vi "Test - Draw Teapot.vi"() -> ()   [LabVIEW 2022 SP3, in "Raster.lvlib"] (continued)
"y"=394.73068, "z"=0.98822266}, "UV"={"u"=0.0, "v"=0.0}, "Colour"=12517256}, "Alpha"=0.0, "Alpha Blending Enabled"=FALSE, "Colour"=8630366}, {"Vertex 1"={"Position"={"x"=469.49927, "y"=102.06894, "z"=0.9882263}, "UV"={"u"=0.0, "v"=0.0}, "Colour"=12517256}, "Vertex 2"={"Position"={"x"=448.97742, "y"=109.926476, "z"=0.9887645}, "UV"={"u"=0.0, "v"=0.0}, "Colour"=12517256}, "Vertex 3"={"Position"={"x"=438.67215, "y"=107.464905, "z"=0.9886184}, "UV"={"u"=0.0, "v"=0.0}, "Colour"=12517256}, "Alpha"=0.0, "Alpha Blending Enabled"=FALSE, "Colour"=131841}, {"Vertex 1"={"Position"={"x"=353.4767, "y"=412.15842, "z"=0.988328}, "UV"={"u"=0.0, "v"=0.0}, "Colour"=12517256}, "Vertex 2"={"Position"={"x"=363.17734, "y"=411.41696, "z"=0.9886868}, "UV"={"u"=0.0, "v"=0.0}, "Colour"=12517256}, "Vertex 3"={"Position"={"x"=374.3895, "y"=412.44833, "z"=0.98858166}, "UV"={"u"=0.0, "v"=0.0}, "Colour"=12517256}, "Alpha"=0.0, "Alpha Blending Enabled"=FALSE, "Colour"=9948012}, {"Vertex 1"={"Position"={"x"=272.53372, "y"=105.9543, "z"=0.9882486}, "UV"={"u"=0.0, "v"=0.0}, "Colour"=12517256}, "Vertex 2"={"Position"={"x"=288.70093, "y"=107.824104, "z"=0.9884769}, "UV"={"u"=0.0, "v"=0.0}, "Colour"=12517256}, "Vertex 3"={"Position"={"x"=281.7214, "y"=114.2621, "z"=0.98886466}, "UV"={"u"=0.0, "v"=0.0}, "Colour"=12517256}, "Alpha"=0.0, "Alpha Blending Enabled"=FALSE, "Colour"=131841}, {"Vertex 1"={"Position"={"x"=567.6066, "y"=128.19644, "z"=0.98837066}, "UV"={"u"=0.0, "v"=0.0}, "Colour"=12517256}, "Vertex 2"={"Position"={"x"=574.71216, "y"=132.81842, "z"=0.9882995}, "UV"={"u"=0.0, "v"=0.0}, "Colour"=12517256}, "Vertex 3"={"Position"={"x"=576.8591, "y"=141.4411, "z"=0.98890555}, "UV"={"u"=0.0, "v"=0.0}, "Colour"=12517256}, "Alpha"=0.0, "Alpha Blending Enabled"=FALSE, "Colour"=131841}, {"Vertex 1"={"Position"={"x"=193.75427, "y"=299.13568, "z"=0.9887155}, "UV"={"u"=0.0, "v"=0.0}, "Colour"=12517256}, "Vertex 2"={"Position"={"x"=201.29657, "y"=317.0733, "z"=0.9887643}, "UV"={"u"=0.0, "v"=0.0}, "Colour"=12517256}, "Vertex 3"={"Position"={"x"=202.38127, "y"=318.1235, "z"=0.98807013}, "UV"={"u"=0.0, "v"=0.0}, "Colour"=12517256}, "Alpha"=0.0, "Alpha Blending Enabled"=FALSE, "Colour"=6390341}, {"Vertex 1"={"Position"={"x"=205.55954, "y"=154.37106, "z"=0.98879194}, "UV"={"u"=0.0, "v"=0.0}, "Colour"=12517256}, "Vertex 2"={"Position"={"x"=196.25456, "y"=162.86359, "z"=0.98873174}, "UV"={"u"=0.0, "v"=0.0}, "Colour"=12517256}, "Vertex 3"={"Position"={"x"=197.05006, "y"=154.20059, "z"=0.9880167}, "UV"={"u"=0.0, "v"=0.0}, "Colour"=12517256}, "Alpha"=0.0, "Alpha Blending Enabled"=FALSE, "Colour"=131841}, {"Vertex 1"={"Position"={"x"=546.60223, "y"=113.55681, "z"=0.98858106}, "UV"={"u"=0.0, "v"=0.0}, "Colour"=12517256}, "Vertex 2"={"Position"={"x"=534.80365, "y"=113.363174, "z"=0.98869914}, "UV"={"u"=0.0, "v"=0.0}, "Colour"=12517256}, "Vertex 3"={"Position"={"x"=527.4663, "y"=105.9543, "z"=0.9882486}, "UV"={"u"=0.0, "v"=0.0}, "Colour"=12517256}, "Alpha"=0.0, "Alpha Blending Enabled"=FALSE, "Colour"=131841}, {"Vertex 1"={"Position"={"x"=363.17734, "y"=411.41696, "z"=0.9886868}, "UV"={"u"=0.0, "v"=0.0}, "Colour"=12517256}, "Vertex 2"={"Position"={"x"=353.4767, "y"=412.15842, "z"=0.988328}, "UV"={"u"=0.0, "v"=0.0}, "Colour"=12517256}, "Vertex 3"={"Position"={"x"=341.23203, "y"=410.43784, "z"=0.98850775}, "UV"={"u"=0.0, "v"=0.0}, "Colour"=12517256}, "Alpha"=0.0, "Alpha Blending Enabled"=FALSE, "Colour"=9881963}, {"Vertex 1"={"Position"={"x"=579.84076, "y"=355.96957, "z"=0.98824817}, "UV"={"u"=0.0, "v"=0.0}, "Colour"=12517256}, "Vertex 2"={"Position"={"x"=570.48285, "y"=374.62314, "z"=0.98834187}, "UV"={"u"=0.0, "v"=0.0}, "Colour"=12517256}, "Vertex 3"={"Position"={"x"=572.7935, "y"=370.8628, "z"=0.98893183}, "UV"={"u"=0.0, "v"=0.0}, "Colour"=12517256}, "Alpha"=0.0, "Alpha Blending Enabled"=FALSE, "Colour"=6851402}, {"Vertex 1"={"Position"={"x"=492.24643, "y"=405.47995, "z"=0.98874605}, "UV"={"u"=0.0, "v"=0.0}, "Colour"=12517256}, "Vertex 2"={"Position"={"x"=506.44025, "y"=404.4099, "z"=0.98854554}, "UV"={"u"=0.0, "v"=0.0}, "Colour"=12517256}, "Vertex 3"={"Position"={"x"=496.2093, "y"=407.57056, "z"=0.9881973}, "UV"={"u"=0.0, "v"=0.0}, "Colour"=12517256}, "Alpha"=0.0, "Alpha Blending Enabled"=FALSE, "Colour"=9750378}, {"Vertex 1"={"Position"={"x"=448.97742, "y"=109.926476, "z"=0.9887645}, "UV"={"u"=0.0, "v"=0.0}, "Colour"=12517256}, "Vertex 2"={"Position"={"x"=469.49927, "y"=102.06894, "z"=0.9882263}, "UV"={"u"=0.0, "v"=0.0}, "Colour"=12517256}, "Vertex 3"={"Position"={"x"=481.26578, "y"=106.39749, "z"=0.9884849}, "UV"={"u"=0.0, "v"=0.0}, "Colour"=12517256}, "Alpha"=0.0, "Alpha Blending Enabled"=FALSE, "Colour"=131841}, {"Vertex 1"={"Position"={"x"=598.7034, "y"=317.0733, "z"=0.9887643}, "UV"={"u"=0.0, "v"=0.0}, "Colour"=12517256}, "Vertex 2"={"Position"={"x"=606.2457, "y"=299.13568, "z"=0.9887155}, "UV"={"u"=0.0, "v"=0.0}, "Colour"=12517256}, "Vertex 3"={"Position"={"x"=605.6, "y"=299.08035, "z"=0.98799026}, "UV"={"u"=0.0, "v"=0.0}, "Colour"=12517256}, "Alpha"=0.0, "Alpha Blending Enabled"=FALSE, "Colour"=6390341}, {"Vertex 1"={"Position"={"x"=229.51718, "y"=374.62314, "z"=0.98834187}, "UV"={"u"=0.0, "v"=0.0}, "Colour"=12517256}, "Vertex 2"={"Position"={"x"=220.15924, "y"=355.96957, "z"=0.98824817}, "UV"={"u"=0.0, "v"=0.0}, "Colour"=12517256}, "Vertex 3"={"Position"={"x"=218.2245, "y"=353.0026, "z"=0.9888737}, "UV"={"u"=0.0, "v"=0.0}, "Colour"=12517256}, "Alpha"=0.0, "Alpha Blending Enabled"=FALSE, "Colour"=6851402}, {"Vertex 1"={"Position"={"x"=432.43652, "y"=413.4734, "z"=0.9881905}, "UV"={"u"=0.0, "v"=0.0}, "Colour"=12517256}, "Vertex 2"={"Position"={"x"=425.6105, "y"=412.44833, "z"=0.98858166}, "UV"={"u"=0.0, "v"=0.0}, "Colour"=12517256}, "Vertex 3"={"Position"={"x"=436.8227, "y"=411.41696, "z"=0.9886868}, "UV"={"u"=0.0, "v"=0.0}, "Colour"=12517256}, "Alpha"=0.0, "Alpha Blending Enabled"=FALSE, "Colour"=9948012}, {"Vertex 1"={"Position"={"x"=526.323, "y"=399.39044, "z"=0.9882647}, "UV"={"u"=0.0, "v"=0.0}, "Colour"=12517256}, "Vertex 2"={"Position"={"x"=518.25006, "y"=402.50375, "z"=0.98837876}, "UV"={"u"=0.0, "v"=0.0}, "Colour"=12517256}, "Vertex 3"={"Position"={"x"=525.403, "y"=398.86298, "z"=0.98879325}, "UV"={"u"=0.0, "v"=0.0}, "Colour"=12517256}, "Alpha"=0.0, "Alpha Blending Enabled"=FALSE, "Colour"=10013549}, {"Vertex 1"={"Position"={"x"=511.29907, "y"=107.824104, "z"=0.9884769}, "UV"={"u"=0.0, "v"=0.0}, "Colour"=12517256}, "Vertex 2"={"Position"={"x"=527.4663, "y"=105.9543, "z"=0.9882486}, "UV"={"u"=0.0, "v"=0.0}, "Colour"=12517256}, "Vertex 3"={"Position"={"x"=534.80365, "y"=113.363174, "z"=0.98869914}, "UV"={"u"=0.0, "v"=0.0}, "Colour"=12517256}, "Alpha"=0.0, "Alpha Blending Enabled"=FALSE, "Colour"=131841}, {"Vertex 1"={"Position"={"x"=612.38416, "y"=172.88614, "z"=0.98867583}, "UV"={"u"=0.0, "v"=0.0}, "Colour"=12517256}, "Vertex 2"={"Position"={"x"=603.7455, "y"=162.86359, "z"=0.98873174}, "UV"={"u"=0.0, "v"=0.0}, "Colour"=12517256}, "Vertex 3"={"Position"={"x"=602.9499, "y"=154.20059, "z"=0.9880167}, "UV"={"u"=0.0, "v"=0.0}, "Colour"=12517256}, "Alpha"=0.0, "Alpha Blending Enabled"=FALSE, "Colour"=131841}, {"Vertex 1"={"Position"={"x"=216.54234, "y"=138.55649, "z"=0.9882119}, "UV"={"u"=0.0, "v"=0.0}, "Colour"=12517256}, "Vertex 2"={"Position"={"x"=225.2878, "y"=132.81842, "z"=0.9882995}, "UV"={"u"=0.0, "v"=0.0}, "Colour"=12517256}, "Vertex 3"={"Position"={"x"=223.14096, "y"=141.4411, "z"=0.98890555}, "UV"={"u"=0.0, "v"=0.0}, "Colour"=12517256}, "Alpha"=0.0, "Alpha Blending Enabled"=FALSE, "Colour"=131841}, {"Vertex 1"={"Position"={"x"=471.05533, "y"=410.71017, "z"=0.9881855}, "UV"={"u"=0.0, "v"=0.0}, "Colour"=12517256}, "Vertex 2"={"Position"={"x"=458.76797, "y"=410.43784, "z"=0.98850775}, "UV"={"u"=0.0, "v"=0.0}, "Colour"=12517256}, "Vertex 3"={"Position"={"x"=468.95047, "y"=408.38864, "z"=0.98872197}, "UV"={"u"=0.0, "v"=0.0}, "Colour"=12517256}, "Alpha"=0.0, "Alpha Blending Enabled"=FALSE, "Colour"=9815914}, {"Vertex 1"={"Position"={"x"=496.2093, "y"=407.57056, "z"=0.9881973}, "UV"={"u"=0.0, "v"=0.0}, "Colour"=12517256}, "Vertex 2"={"Position"={"x"=483.04462, "y"=408.23608, "z"=0.98845065}, "UV"={"u"=0.0, "v"=0.0}, "Colour"=12517256}, "Vertex 3"={"Position"={"x"=492.24643, "y"=405.47995, "z"=0.98874605}, "UV"={"u"=0.0, "v"=0.0}, "Colour"=12517256}, "Alpha"=0.0, "Alpha Blending Enabled"=FALSE, "Colour"=9750378}, {"Vertex 1"={"Position"={"x"=344.82437, "y"=98.41171, "z"=0.9880079}, "UV"={"u"=0.0, "v"=0.0}, "Colour"=12517256}, "Vertex 2"={"Position"={"x"=361.32785, "y"=107.464905, "z"=0.9886184}, "UV"={"u"=0.0, "v"=0.0}, "Colour"=12517256}, "Vertex 3"={"Position"={"x"=351.02258, "y"=109.926476, "z"=0.9887645}, "UV"={"u"=0.0, "v"=0.0}, "Colour"=12517256}, "Alpha"=0.0, "Alpha Blending Enabled"=FALSE, "Colour"=131841}, {"Vertex 1"={"Position"={"x"=187.10504, "y"=281.3187, "z"=0.9886726}, "UV"={"u"=0.0, "v"=0.0}, "Colour"=12517256}, "Vertex 2"={"Position"={"x"=193.75427, "y"=299.13568, "z"=0.9887155}, "UV"={"u"=0.0, "v"=0.0}, "Colour"=12517256}, "Vertex 3"={"Position"={"x"=194.40005, "y"=299.08035, "z"=0.98799026}, "UV"={"u"=0.0, "v"=0.0}, "Colour"=12517256}, "Alpha"=0.0, "Alpha Blending Enabled"=FALSE, "Colour"=6126914}, {"Vertex 1"={"Position"={"x"=299.2597, "y"=101.732666, "z"=0.98811007}, "UV"={"u"=0.0, "v"=0.0}, "Colour"=12517256}, "Vertex 2"={"Position"={"x"=318.7342, "y"=106.39749, "z"=0.9884849}, "UV"={"u"=0.0, "v"=0.0}, "Colour"=12517256}, "Vertex 3"={"Position"={"x"=309.68015, "y"=111.224434, "z"=0.9887732}, "UV"={"u"=0.0, "v"=0.0}, "Colour"=12517256}, "Alpha"=0.0, "Alpha Blending Enabled"=FALSE, "Colour"=131841}, {"Vertex 1"={"Position"={"x"=265.19638, "y"=113.363174, "z"=0.98869914}, "UV"={"u"=0.0, "v"=0.0}, "Colour"=12517256}, "Vertex 2"={"Position"={"x"=253.39772, "y"=113.55681, "z"=0.98858106}, "UV"={"u"=0.0, "v"=0.0}, "Colour"=12517256}, "Vertex 3"={"Position"={"x"=260.89398, "y"=105.47977, "z"=0.9880842}, "UV"={"u"=0.0, "v"=0.0}, "Colour"=12517256}, "Alpha"=0.0, "Alpha Blending Enabled"=FALSE, "Colour"=131841}, {"Vertex 1"={"Position"={"x"=574.71216, "y"=132.81842, "z"=0.9882995}, "UV"={"u"=0.0, "v"=0.0}, "Colour"=12517256}, "Vertex 2"={"Position"={"x"=583.45764, "y"=138.55649, "z"=0.9882119}, "UV"={"u"=0.0, "v"=0.0}, "Colour"=12517256}, "Vertex 3"={"Position"={"x"=585.23376, "y"=147.27748, "z"=0.9888514}, "UV"={"u"=0.0, "v"=0.0}, "Colour"=12517256}, "Alpha"=0.0, "Alpha Blending Enabled"=FALSE, "Colour"=131841}, {"Vertex 1"={"Position"={"x"=309.68015, "y"=111.224434, "z"=0.9887732}, "UV"={"u"=0.0, "v"=0.0}, "Colour"=12517256}, "Vertex 2"={"Position"={"x"=288.70093, "y"=107.824104, "z"=0.9884769}, "UV"={"u"=0.0, "v"=0.0}, "Colour"=12517256}, "Vertex 3"={"Position"={"x"=299.2597, "y"=101.732666, "z"=0.98811007}, "UV"={"u"=0.0, "v"=0.0}, "Colour"=12517256}, "Alpha"=0.0, "Alpha Blending Enabled"=FALSE, "Colour"=131841}, {"Vertex 1"={"Position"={"x"=468.95047, "y"=408.38864, "z"=0.98872197}, "UV"={"u"=0.0, "v"=0.0}, "Colour"=12517256}, "Vertex 2"={"Position"={"x"=483.04462, "y"=408.23608, "z"=0.98845065}, "UV"={"u"=0.0, "v"=0.0}, "Colour"=12517256}, "Vertex 3"={"Position"={"x"=471.05533, "y"=410.71017, "z"=0.9881855}, "UV"={"u"=0.0, "v"=0.0}, "Colour"=12517256}, "Alpha"=0.0, "Alpha Blending Enabled"=FALSE, "Colour"=9815914}, {"Vertex 1"={"Position"={"x"=281.74997, "y"=402.50375, "z"=0.98837876}, "UV"={"u"=0.0, "v"=0.0}, "Colour"=12517256}, "Vertex 2"={"Position"={"x"=273.677, "y"=399.39044, "z"=0.9882647}, "UV"={"u"=0.0, "v"=0.0}, "Colour"=12517256}, "Vertex 3"={"Position"={"x"=266.35956, "y"=395.62842, "z"=0.98871076}, "UV"={"u"=0.0, "v"=0.0}, "Colour"=12517256}, "Alpha"=0.0, "Alpha Blending Enabled"=FALSE, "Colour"=10013549}, {"Vertex 1"={"Position"={"x"=196.25456, "y"=162.86359, "z"=0.98873174}, "UV"={"u"=0.0, "v"=0.0}, "Colour"=12517256}, "Vertex 2"={"Position"={"x"=187.61583, "y"=172.88614, "z"=0.98867583}, "UV"={"u"=0.0, "v"=0.0}, "Colour"=12517256}, "Vertex 3"={"Position"={"x"=187.87697, "y"=164.49333, "z"=0.9879249}, "UV"={"u"=0.0, "v"=0.0}, "Colour"=12517256}, "Alpha"=0.0, "Alpha Blending Enabled"=FALSE, "Colour"=131841}, {"Vertex 1"={"Position"={"x"=606.2457, "y"=299.13568, "z"=0.9887155}, "UV"={"u"=0.0, "v"=0.0}, "Colour"=12517256}, "Vertex 2"={"Position"={"x"=612.89496, "y"=281.3187, "z"=0.9886726}, "UV"={"u"=0.0, "v"=0.0}, "Colour"=12517256}, "Vertex 3"={"Position"={"x"=612.6671, "y"=280.0821, "z"=0.98791945}, "UV"={"u"=0.0, "v"=0.0}, "Colour"=12517256}, "Alpha"=0.0, "Alpha Blending Enabled"=FALSE, "Colour"=6126914}, {"Vertex 1"={"Position"={"x"=367.56348, "y"=413.4734, "z"=0.9881905}, "UV"={"u"=0.0, "v"=0.0}, "Colour"=12517256}, "Vertex 2"={"Position"={"x"=374.3895, "y"=412.44833, "z"=0.98858166}, "UV"={"u"=0.0, "v"=0.0}, "Colour"=12517256}, "Vertex 3"={"Position"={"x"=386.75226, "y"=413.1011, "z"=0.988515}, "UV"={"u"=0.0, "v"=0.0}, "Colour"=12517256}, "Alpha"=0.0, "Alpha Blending Enabled"=FALSE, "Colour"=10013805}, {"Vertex 1"={"Position"={"x"=588.9574, "y"=337.11398, "z"=0.98815686}, "UV"={"u"=0.0, "v"=0.0}, "Colour"=12517256}, "Vertex 2"={"Position"={"x"=579.84076, "y"=355.96957, "z"=0.98824817}, "UV"={"u"=0.0, "v"=0.0}, "Colour"=12517256}, "Vertex 3"={"Position"={"x"=581.77545, "y"=353.0026, "z"=0.9888737}, "UV"={"u"=0.0, "v"=0.0}, "Colour"=12517256}, "Alpha"=0.0, "Alpha Blending Enabled"=FALSE, "Colour"=6719817}, {"Vertex 1"={"Position"={"x"=619.56256, "y"=184.55232, "z"=0.98862946}, "UV"={"u"=0.0, "v"=0.0}, "Colour"=12517256}, "Vertex 2"={"Position"={"x"=612.38416, "y"=172.88614, "z"=0.98867583}, "UV"={"u"=0.0, "v"=0.0}, "Colour"=12517256}, "Vertex 3"={"Position"={"x"=612.123, "y"=164.49333, "z"=0.9879249}, "UV"={"u"=0.0, "v"=0.0}, "Colour"=12517256}, "Alpha"=0.0, "Alpha Blending Enabled"=FALSE, "Colour"=131841}, {"Vertex 1"={"Position"={"x"=181.5629, "y"=263.7103, "z"=0.98863673}, "UV"={"u"=0.0, "v"=0.0}, "Colour"=12517256}, "Vertex 2"={"Position"={"x"=187.10504, "y"=281.3187, "z"=0.9886726}, "UV"={"u"=0.0, "v"=0.0}, "Colour"=12517256}, "Vertex 3"={"Position"={"x"=187.33292, "y"=280.0821, "z"=0.98791945}, "UV"={"u"=0.0, "v"=0.0}, "Colour"=12517256}, "Alpha"=0.0, "Alpha Blending Enabled"=FALSE, "Colour"=5731646}, {"Vertex 1"={"Position"={"x"=220.15924, "y"=355.96957, "z"=0.98824817}, "UV"={"u"=0.0, "v"=0.0}, "Colour"=12517256}, "Vertex 2"={"Position"={"x"=211.0426, "y"=337.11398, "z"=0.98815686}, "UV"={"u"=0.0, "v"=0.0}, "Colour"=12517256}, "Vertex 3"={"Position"={"x"=209.52173, "y"=335.05237, "z"=0.9888175}, "UV"={"u"=0.0, "v"=0.0}, "Colour"=12517256}, "Alpha"=0.0, "Alpha Blending Enabled"=FALSE, "Colour"=6719817}, {"Vertex 1"={"Position"={"x"=436.8227, "y"=411.41696, "z"=0.9886868}, "UV"={"u"=0.0, "v"=0.0}, "Colour"=12517256}, "Vertex 2"={"Position"={"x"=446.5233, "y"=412.15842, "z"=0.988328}, "UV"={"u"=0.0, "v"=0.0}, "Colour"=12517256}, "Vertex 3"={"Position"={"x"=432.43652, "y"=413.4734, "z"=0.9881905}, "UV"={"u"=0.0, "v"=0.0}, "Colour"=12517256}, "Alpha"=0.0, "Alpha Blending Enabled"=FALSE, "Colour"=9948012}, {"Vertex 1"={"Position"={"x"=416.8047, "y"=414.309, "z"=0.98810315}, "UV"={"u"=0.0, "v"=0.0}, "Colour"=12517256}, "Vertex 2"={"Position"={"x"=413.24774, "y"=413.1011, "z"=0.988515}, "UV"={"u"=0.0, "v"=0.0}, "Colour"=12517256}, "Vertex 3"={"Position"={"x"=425.6105, "y"=412.44833, "z"=0.98858166}, "UV"={"u"=0.0, "v"=0.0}, "Colour"=12517256}, "Alpha"=0.0, "Alpha Blending Enabled"=FALSE, "Colour"=10013805}, {"Vertex 1"={"Position"={"x"=529.3001, "y"=394.73068, "z"=0.98822266}, "UV"={"u"=0.0, "v"=0.0}, "Colour"=12517256}, "Vertex 2"={"Position"={"x"=526.323, "y"=399.39044, "z"=0.9882647}, "UV"={"u"=0.0, "v"=0.0}, "Colour"=12517256}, "Vertex 3"={"Position"={"x"=533.64044, "y"=395.62842, "z"=0.98871076}, "UV"={"u"=0.0, "v"=0.0}, "Colour"=12517256}, "Alpha"=0.0, "Alpha Blending Enabled"=FALSE, "Colour"=8630366}, {"Vertex 1"={"Position"={"x"=316.9554, "y"=408.23608, "z"=0.98845065}, "UV"={"u"=0.0, "v"=0.0}, "Colour"=12517256}, "Vertex 2"={"Position"={"x"=303.7907, "y"=407.57056, "z"=0.9881973}, "UV"={"u"=0.0, "v"=0.0}, "Colour"=12517256}, "Vertex 3"={"Position"={"x"=293.55975, "y"=404.4099, "z"=0.98854554}, "UV"={"u"=0.0, "v"=0.0}, "Colour"=12517256}, "Alpha"=0.0, "Alpha Blending Enabled"=FALSE, "Colour"=9750378}, {"Vertex 1"={"Position"={"x"=206.8759, "y"=145.61699, "z"=0.9881152}, "UV"={"u"=0.0, "v"=0.0}, "Colour"=12517256}, "Vertex 2"={"Position"={"x"=216.54234, "y"=138.55649, "z"=0.9882119}, "UV"={"u"=0.0, "v"=0.0}, "Colour"=12517256}, "Vertex 3"={"Position"={"x"=214.76619, "y"=147.27748, "z"=0.9888514}, "UV"={"u"=0.0, "v"=0.0}, "Colour"=12517256}, "Alpha"=0.0, "Alpha Blending Enabled"=FALSE, "Colour"=131841}, {"Vertex 1"={"Position"={"x"=612.89496, "y"=281.3187, "z"=0.9886726}, "UV"={"u"=0.0, "v"=0.0}, "Colour"=12517256}, "Vertex 2"={"Position"={"x"=618.4371, "y"=263.7103, "z"=0.98863673}, "UV"={"u"=0.0, "v"=0.0}, "Colour"=12517256}, "Vertex 3"={"Position"={"x"=618.57983, "y"=261.2413, "z"=0.9878602}, "UV"={"u"=0.0, "v"=0.0}, "Colour"=12517256}, "Alpha"=0.0, "Alpha Blending Enabled"=FALSE, "Colour"=5731646}, {"Vertex 1"={"Position"={"x"=554.3064, "y"=114.66924, "z"=0.9885038}, "UV"={"u"=0.0, "v"=0.0}, "Colour"=12517256}, "Vertex 2"={"Position"={"x"=546.60223, "y"=113.55681, "z"=0.98858106}, "UV"={"u"=0.0, "v"=0.0}, "Colour"=12517256}, "Vertex 3"={"Position"={"x"=539.10596, "y"=105.47977, "z"=0.9880842}, "UV"={"u"=0.0, "v"=0.0}, "Colour"=12517256}, "Alpha"=0.0, "Alpha Blending Enabled"=FALSE, "Colour"=131841}, {"Vertex 1"={"Position"={"x"=273.677, "y"=399.39044, "z"=0.9882647}, "UV"={"u"=0.0, "v"=0.0}, "Colour"=12517256}, "Vertex 2"={"Position"={"x"=270.6999, "y"=394.73068, "z"=0.98822266}, "UV"={"u"=0.0, "v"=0.0}, "Colour"=12517256}, "Vertex 3"={"Position"={"x"=263.33197, "y"=391.06378, "z"=0.9886805}, "UV"={"u"=0.0, "v"=0.0}, "Colour"=12517256}, "Alpha"=0.0, "Alpha Blending Enabled"=FALSE, "Colour"=8630366}, {"Vertex 1"={"Position"={"x"=187.61583, "y"=172.88614, "z"=0.98867583}, "UV"={"u"=0.0, "v"=0.0}, "Colour"=12517256}, "Vertex 2"={"Position"={"x"=180.43742, "y"=184.55232, "z"=0.98862946}, "UV"={"u"=0.0, "v"=0.0}, "Colour"=12517256}, "Vertex 3"={"Position"={"x"=180.21684, "y"=176.65451, "z"=0.98784816}, "UV"={"u"=0.0, "v"=0.0}, "Colour"=12517256}, "Alpha"=0.0, "Alpha Blending Enabled"=FALSE, "Colour"=131841}, {"Vertex 1"={"Position"={"x"=341.23203, "y"=410.43784, "z"=0.98850775}, "UV"={"u"=0.0, "v"=0.0}, "Colour"=12517256}, "Vertex 2"={"Position"={"x"=328.94467, "y"=410.71017, "z"=0.9881855}, "UV"={"u"=0.0, "v"=0.0}, "Colour"=12517256}, "Vertex 3"={"Position"={"x"=316.9554, "y"=408.23608, "z"=0.98845065}, "UV"={"u"=0.0, "v"=0.0}, "Colour"=12517256}, "Alpha"=0.0, "Alpha Blending Enabled"=FALSE, "Colour"=9815914}, {"Vertex 1"={"Position"={"x"=248.83113, "y"=403.53403, "z"=0.9885353}, "UV"={"u"=0.0, "v"=0.0}, "Colour"=12517256}, "Vertex 2"={"Position"={"x"=250.87166, "y"=403.82065, "z"=0.98855567}, "UV"={"u"=0.0, "v"=0.0}, "Colour"=12517256}, "Vertex 3"={"Position"={"x"=258.39148, "y"=408.39923, "z"=0.9880488}, "UV"={"u"=0.0, "v"=0.0}, "Colour"=12517256}, "Alpha"=0.0, "Alpha Blending Enabled"=FALSE, "Colour"=9684329}, {"Vertex 1"={"Position"={"x"=455.17563, "y"=98.41171, "z"=0.9880079}, "UV"={"u"=0.0, "v"=0.0}, "Colour"=12517256}, "Vertex 2"={"Position"={"x"=438.67215, "y"=107.464905, "z"=0.9886184}, "UV"={"u"=0.0, "v"=0.0}, "Colour"=12517256}, "Vertex 3"={"Position"={"x"=426.90945, "y"=105.592224, "z"=0.9885072}, "UV"={"u"=0.0, "v"=0.0}, "Colour"=12517256}, "Alpha"=0.0, "Alpha Blending Enabled"=FALSE, "Colour"=131841}, {"Vertex 1"={"Position"={"x"=281.74997, "y"=402.50375, "z"=0.98837876}, "UV"={"u"=0.0, "v"=0.0}, "Colour"=12517256}, "Vertex 2"={"Position"={"x"=293.55975, "y"=404.4099, "z"=0.98854554}, "UV"={"u"=0.0, "v"=0.0}, "Colour"=12517256}, "Vertex 3"={"Position"={"x"=303.7907, "y"=407.57056, "z"=0.9881973}, "UV"={"u"=0.0, "v"=0.0}, "Colour"=12517256}, "Alpha"=0.0, "Alpha Blending Enabled"=FALSE, "Colour"=10014061}, {"Vertex 1"={"Position"={"x"=583.45764, "y"=138.55649, "z"=0.9882119}, "UV"={"u"=0.0, "v"=0.0}, "Colour"=12517256}, "Vertex 2"={"Position"={"x"=593.1241, "y"=145.61699, "z"=0.9881152}, "UV"={"u"=0.0, "v"=0.0}, "Colour"=12517256}, "Vertex 3"={"Position"={"x"=594.4404, "y"=154.37106, "z"=0.98879194}, "UV"={"u"=0.0, "v"=0.0}, "Colour"=12517256}, "Alpha"=0.0, "Alpha Blending Enabled"=FALSE, "Colour"=131841}, {"Vertex 1"={"Position"={"x"=549.12836, "y"=403.82065, "z"=0.98855567}, "UV"={"u"=0.0, "v"=0.0}, "Colour"=12517256}, "Vertex 2"={"Position"={"x"=551.1689, "y"=403.53403, "z"=0.9885353}, "UV"={"u"=0.0, "v"=0.0}, "Colour"=12517256}, "Vertex 3"={"Position"={"x"=543.6329, "y"=408.16522, "z"=0.9880202}, "UV"={"u"=0.0, "v"=0.0}, "Colour"=12517256}, "Alpha"=0.0, "Alpha Blending Enabled"=FALSE, "Colour"=9684329}, {"Vertex 1"={"Position"={"x"=383.19528, "y"=414.309, "z"=0.98810315}, "UV"={"u"=0.0, "v"=0.0}, "Colour"=12517256}, "Vertex 2"={"Position"={"x"=386.75226, "y"=413.1011, "z"=0.988515}, "UV"={"u"=0.0, "v"=0.0}, "Colour"=12517256}, "Vertex 3"={"Position"={"x"=400.0, "y"=413.3279, "z"=0.9884919}, "UV"={"u"=0.0, "v"=0.0}, "Colour"=12517256}, "Alpha"=0.0, "Alpha Blending Enabled"=FALSE, "Colour"=10079597}, {"Vertex 1"={"Position"={"x"=177.34291, "y"=246.40646, "z"=0.98860943}, "UV"={"u"=0.0, "v"=0.0}, "Colour"=12517256}, "Vertex 2"={"Position"={"x"=181.5629, "y"=263.7103, "z"=0.98863673}, "UV"={"u"=0.0, "v"=0.0}, "Colour"=12517256}, "Vertex 3"={"Position"={"x"=181.4201, "y"=261.2413, "z"=0.9878602}, "UV"={"u"=0.0, "v"=0.0}, "Colour"=12517256}, "Alpha"=0.0, "Alpha Blending Enabled"=FALSE, "Colour"=5270329}, {"Vertex 1"={"Position"={"x"=374.3895, "y"=412.44833, "z"=0.98858166}, "UV"={"u"=0.0, "v"=0.0}, "Colour"=12517256}, "Vertex 2"={"Position"={"x"=367.56348, "y"=413.4734, "z"=0.9881905}, "UV"={"u"=0.0, "v"=0.0}, "Colour"=12517256}, "Vertex 3"={"Position"={"x"=353.4767, "y"=412.15842, "z"=0.988328}, "UV"={"u"=0.0, "v"=0.0}, "Colour"=12517256}, "Alpha"=0.0, "Alpha Blending Enabled"=FALSE, "Colour"=9948012}, {"Vertex 1"={"Position"={"x"=400.0, "y"=414.5999, "z"=0.98807275}, "UV"={"u"=0.0, "v"=0.0}, "Colour"=12517256}, "Vertex 2"={"Position"={"x"=400.0, "y"=413.3279, "z"=0.9884919}, "UV"={"u"=0.0, "v"=0.0}, "Colour"=12517256}, "Vertex 3"={"Position"={"x"=413.24774, "y"=413.1011, "z"=0.988515}, "UV"={"u"=0.0, "v"=0.0}, "Colour"=12517256}, "Alpha"=0.0, "Alpha Blending Enabled"=FALSE, "Colour"=10079597}, {"Vertex 1"={"Position"={"x"=624.4671, "y"=197.94992, "z"=0.98859775}, "UV"={"u"=0.0, "v"=0.0}, "Colour"=12517256}, "Vertex 2"={"Position"={"x"=619.56256, "y"=184.55232, "z"=0.98862946}, "UV"={"u"=0.0, "v"=0.0}, "Colour"=12517256}, "Vertex 3"={"Position"={"x"=619.78314, "y"=176.65451, "z"=0.98784816}, "UV"={"u"=0.0, "v"=0.0}, "Colour"=12517256}, "Alpha"=0.0, "Alpha Blending Enabled"=FALSE, "Colour"=461061}, {"Vertex 1"={"Position"={"x"=481.26578, "y"=106.39749, "z"=0.9884849}, "UV"={"u"=0.0, "v"=0.0}, "Colour"=12517256}, "Vertex 2"={"Position"={"x"=500.7403, "y"=101.732666, "z"=0.98811007}, "UV"={"u"=0.0, "v"=0.0}, "Colour"=12517256}, "Vertex 3"={"Position"={"x"=511.29907, "y"=107.824104, "z"=0.9884769}, "UV"={"u"=0.0, "v"=0.0}, "Colour"=12517256}, "Alpha"=0.0, "Alpha Blending Enabled"=FALSE, "Colour"=131841}, {"Vertex 1"={"Position"={"x"=246.46959, "y"=402.33032, "z"=0.9885116}, "UV"={"u"=0.0, "v"=0.0}, "Colour"=12517256}, "Vertex 2"={"Position"={"x"=248.83113, "y"=403.53403, "z"=0.9885353}, "UV"={"u"=0.0, "v"=0.0}, "Colour"=12517256}, "Vertex 3"={"Position"={"x"=256.36713, "y"=408.16522, "z"=0.9880202}, "UV"={"u"=0.0, "v"=0.0}, "Colour"=12517256}, "Alpha"=0.0, "Alpha Blending Enabled"=FALSE, "Colour"=9948012}, {"Vertex 1"={"Position"={"x"=253.39772, "y"=113.55681, "z"=0.98858106}, "UV"={"u"=0.0, "v"=0.0}, "Colour"=12517256}, "Vertex 2"={"Position"={"x"=245.69356, "y"=114.66924, "z"=0.9885038}, "UV"={"u"=0.0, "v"=0.0}, "Colour"=12517256}, "Vertex 3"={"Position"={"x"=253.24971, "y"=106.19928, "z"=0.9879762}, "UV"={"u"=0.0, "v"=0.0}, "Colour"=12517256}, "Alpha"=0.0, "Alpha Blending Enabled"=FALSE, "Colour"=131841}, {"Vertex 1"={"Position"={"x"=618.4371, "y"=263.7103, "z"=0.98863673}, "UV"={"u"=0.0, "v"=0.0}, "Colour"=12517256}, "Vertex 2"={"Position"={"x"=622.6571, "y"=246.40646, "z"=0.98860943}, "UV"={"u"=0.0, "v"=0.0}, "Colour"=12517256}, "Vertex 3"={"Position"={"x"=623.0958, "y"=242.68484, "z"=0.987815}, "UV"={"u"=0.0, "v"=0.0}, "Colour"=12517256}, "Alpha"=0.0, "Alpha Blending Enabled"=FALSE, "Colour"=5270329}, {"Vertex 1"={"Position"={"x"=597.6187, "y"=318.1235, "z"=0.98807013}, "UV"={"u"=0.0, "v"=0.0}, "Colour"=12517256}, "Vertex 2"={"Position"={"x"=588.9574, "y"=337.11398, "z"=0.98815686}, "UV"={"u"=0.0, "v"=0.0}, "Colour"=12517256}, "Vertex 3"={"Position"={"x"=590.4783, "y"=335.05237, "z"=0.9888175}, "UV"={"u"=0.0, "v"=0.0}, "Colour"=12517256}, "Alpha"=0.0, "Alpha Blending Enabled"=FALSE, "Colour"=6587976}, {"Vertex 1"={"Position"={"x"=551.1689, "y"=403.53403, "z"=0.9885353}, "UV"={"u"=0.0, "v"=0.0}, "Colour"=12517256}, "Vertex 2"={"Position"={"x"=553.5304, "y"=402.33032, "z"=0.9885116}, "UV"={"u"=0.0, "v"=0.0}, "Colour"=12517256}, "Vertex 3"={"Position"={"x"=545.9787, "y"=406.98245, "z"=0.98798704}, "UV"={"u"=0.0, "v"=0.0}, "Colour"=12517256}, "Alpha"=0.0, "Alpha Blending Enabled"=FALSE, "Colour"=9948012}, {"Vertex 1"={"Position"={"x"=260.89398, "y"=105.47977, "z"=0.9880842}, "UV"={"u"=0.0, "v"=0.0}, "Colour"=12517256}, "Vertex 2"={"Position"={"x"=272.53372, "y"=105.9543, "z"=0.9882486}, "UV"={"u"=0.0, "v"=0.0}, "Colour"=12517256}, "Vertex 3"={"Position"={"x"=265.19638, "y"=113.363174, "z"=0.98869914}, "UV"={"u"=0.0, "v"=0.0}, "Colour"=12517256}, "Alpha"=0.0, "Alpha Blending Enabled"=FALSE, "Colour"=131841}, {"Vertex 1"={"Position"={"x"=180.43742, "y"=184.55232, "z"=0.98862946}, "UV"={"u"=0.0, "v"=0.0}, "Colour"=12517256}, "Vertex 2"={"Position"={"x"=175.53291, "y"=197.94992, "z"=0.98859775}, "UV"={"u"=0.0, "v"=0.0}, "Colour"=12517256}, "Vertex 3"={"Position"={"x"=174.96338, "y"=190.80173, "z"=0.9877956}, "UV"={"u"=0.0, "v"=0.0}, "Colour"=12517256}, "Alpha"=0.0, "Alpha Blending Enabled"=FALSE, "Colour"=461061}, {"Vertex 1"={"Position"={"x"=328.94467, "y"=410.71017, "z"=0.9881855}, "UV"={"u"=0.0, "v"=0.0}, "Colour"=12517256}, "Vertex 2"={"Position"={"x"=341.23203, "y"=410.43784, "z"=0.98850775}, "UV"={"u"=0.0, "v"=0.0}, "Colour"=12517256}, "Vertex 3"={"Position"={"x"=353.4767, "y"=412.15842, "z"=0.988328}, "UV"={"u"=0.0, "v"=0.0}, "Colour"=12517256}, "Alpha"=0.0, "Alpha Blending Enabled"=FALSE, "Colour"=9882220}, {"Vertex 1"={"Position"={"x"=174.6588, "y"=229.51056, "z"=0.9885921}, "UV"={"u"=0.0, "v"=0.0}, "Colour"=12517256}, "Vertex 2"={"Position"={"x"=177.34291, "y"=246.40646, "z"=0.98860943}, "UV"={"u"=0.0, "v"=0.0}, "Colour"=12517256}, "Vertex 3"={"Position"={"x"=176.9042, "y"=242.68484, "z"=0.987815}, "UV"={"u"=0.0, "v"=0.0}, "Colour"=12517256}, "Alpha"=0.0, "Alpha Blending Enabled"=FALSE, "Colour"=4677427}, {"Vertex 1"={"Position"={"x"=351.02258, "y"=109.926476, "z"=0.9887645}, "UV"={"u"=0.0, "v"=0.0}, "Colour"=12517256}, "Vertex 2"={"Position"={"x"=330.50076, "y"=102.06894, "z"=0.9882263}, "UV"={"u"=0.0, "v"=0.0}, "Colour"=12517256}, "Vertex 3"={"Position"={"x"=344.82437, "y"=98.41171, "z"=0.9880079}, "UV"={"u"=0.0, "v"=0.0}, "Colour"=12517256}, "Alpha"=0.0, "Alpha Blending Enabled"=FALSE, "Colour"=131841}, {"Vertex 1"={"Position"={"x"=211.0426, "y"=337.11398, "z"=0.98815686}, "UV"={"u"=0.0, "v"=0.0}, "Colour"=12517256}, "Vertex 2"={"Position"={"x"=202.38127, "y"=318.1235, "z"=0.98807013}, "UV"={"u"=0.0, "v"=0.0}, "Colour"=12517256}, "Vertex 3"={"Position"={"x"=201.29657, "y"=317.0733, "z"=0.9887643}, "UV"={"u"=0.0, "v"=0.0}, "Colour"=12517256}, "Alpha"=0.0, "Alpha Blending Enabled"=FALSE, "Colour"=6587976}, {"Vertex 1"={"Position"={"x"=622.6571, "y"=246.40646, "z"=0.98860943}, "UV"={"u"=0.0, "v"=0.0}, "Colour"=12517256}, "Vertex 2"={"Position"={"x"=625.34125, "y"=229.51056, "z"=0.9885921}, "UV"={"u"=0.0, "v"=0.0}, "Colour"=12517256}, "Vertex 3"={"Position"={"x"=625.97455, "y"=224.55252, "z"=0.9877862}, "UV"={"u"=0.0, "v"=0.0}, "Colour"=12517256}, "Alpha"=0.0, "Alpha Blending Enabled"=FALSE, "Colour"=4677427}, {"Vertex 1"={"Position"={"x"=243.93146, "y"=400.19006, "z"=0.9884862}, "UV"={"u"=0.0, "v"=0.0}, "Colour"=12517256}, "Vertex 2"={"Position"={"x"=246.46959, "y"=402.33032, "z"=0.9885116}, "UV"={"u"=0.0, "v"=0.0}, "Colour"=12517256}, "Vertex 3"={"Position"={"x"=254.02132, "y"=406.98245, "z"=0.98798704}, "UV"={"u"=0.0, "v"=0.0}, "Colour"=12517256}, "Alpha"=0.0, "Alpha Blending Enabled"=FALSE, "Colour"=9618536}, {"Vertex 1"={"Position"={"x"=626.281, "y"=213.13216, "z"=0.98858607}, "UV"={"u"=0.0, "v"=0.0}, "Colour"=12517256}, "Vertex 2"={"Position"={"x"=624.4671, "y"=197.94992, "z"=0.98859775}, "UV"={"u"=0.0, "v"=0.0}, "Colour"=12517256}, "Vertex 3"={"Position"={"x"=625.0366, "y"=190.80173, "z"=0.9877956}, "UV"={"u"=0.0, "v"=0.0}, "Colour"=12517256}, "Alpha"=0.0, "Alpha Blending Enabled"=FALSE, "Colour"=2437402}, {"Vertex 1"={"Position"={"x"=361.4469, "y"=95.60257, "z"=0.98784006}, "UV"={"u"=0.0, "v"=0.0}, "Colour"=12517256}, "Vertex 2"={"Position"={"x"=373.09055, "y"=105.592224, "z"=0.9885072}, "UV"={"u"=0.0, "v"=0.0}, "Colour"=12517256}, "Vertex 3"={"Position"={"x"=361.32785, "y"=107.464905, "z"=0.9886184}, "UV"={"u"=0.0, "v"=0.0}, "Colour"=12517256}, "Alpha"=0.0, "Alpha Blending Enabled"=FALSE, "Colour"=131841}, {"Vertex 1"={"Position"={"x"=173.71902, "y"=213.13216, "z"=0.98858607}, "UV"={"u"=0.0, "v"=0.0}, "Colour"=12517256}, "Vertex 2"={"Position"={"x"=174.6588, "y"=229.51056, "z"=0.9885921}, "UV"={"u"=0.0, "v"=0.0}, "Colour"=12517256}, "Vertex 3"={"Position"={"x"=174.02547, "y"=224.55252, "z"=0.9877862}, "UV"={"u"=0.0, "v"=0.0}, "Colour"=12517256}, "Alpha"=0.0, "Alpha Blending Enabled"=FALSE, "Colour"=3886890}, {"Vertex 1"={"Position"={"x"=175.53291, "y"=197.94992, "z"=0.98859775}, "UV"={"u"=0.0, "v"=0.0}, "Colour"=12517256}, "Vertex 2"={"Position"={"x"=173.71902, "y"=213.13216, "z"=0.98858607}, "UV"={"u"=0.0, "v"=0.0}, "Colour"=12517256}, "Vertex 3"={"Position"={"x"=173.01648, "y"=206.9948, "z"=0.9877761}, "UV"={"u"=0.0, "v"=0.0}, "Colour"=12517256}, "Alpha"=0.0, "Alpha Blending Enabled"=FALSE, "Colour"=2437402}, {"Vertex 1"={"Position"={"x"=625.34125, "y"=229.51056, "z"=0.9885921}, "UV"={"u"=0.0, "v"=0.0}, "Colour"=12517256}, "Vertex 2"={"Position"={"x"=626.281, "y"=213.13216, "z"=0.98858607}, "UV"={"u"=0.0, "v"=0.0}, "Colour"=12517256}, "Vertex 3"={"Position"={"x"=626.9835, "y"=206.9948, "z"=0.9877761}, "UV"={"u"=0.0, "v"=0.0}, "Colour"=12517256}, "Alpha"=0.0, "Alpha Blending Enabled"=FALSE, "Colour"=3886890}, {"Vertex 1"={"Position"={"x"=553.5304, "y"=402.33032, "z"=0.9885116}, "UV"={"u"=0.0, "v"=0.0}, "Colour"=12517256}, "Vertex 2"={"Position"={"x"=556.06854, "y"=400.19006, "z"=0.9884862}, "UV"={"u"=0.0, "v"=0.0}, "Colour"=12517256}, "Vertex 3"={"Position"={"x"=548.50366, "y"=404.82367, "z"=0.9879514}, "UV"={"u"=0.0, "v"=0.0}, "Colour"=12517256}, "Alpha"=0.0, "Alpha Blending Enabled"=FALSE, "Colour"=9618536}, {"Vertex 1"={"Position"={"x"=558.6956, "y"=116.502, "z"=0.9884599}, "UV"={"u"=0.0, "v"=0.0}, "Colour"=12517256}, "Vertex 2"={"Position"={"x"=554.3064, "y"=114.66924, "z"=0.9885038}, "UV"={"u"=0.0, "v"=0.0}, "Colour"=12517256}, "Vertex 3"={"Position"={"x"=546.75024, "y"=106.19928, "z"=0.9879762}, "UV"={"u"=0.0, "v"=0.0}, "Colour"=12517256}, "Alpha"=0.0, "Alpha Blending Enabled"=FALSE, "Colour"=131841}, {"Vertex 1"={"Position"={"x"=197.05006, "y"=154.20059, "z"=0.9880167}, "UV"={"u"=0.0, "v"=0.0}, "Colour"=12517256}, "Vertex 2"={"Position"={"x"=206.8759, "y"=145.61699, "z"=0.9881152}, "UV"={"u"=0.0, "v"=0.0}, "Colour"=12517256}, "Vertex 3"={"Position"={"x"=205.55954, "y"=154.37106, "z"=0.98879194}, "UV"={"u"=0.0, "v"=0.0}, "Colour"=12517256}, "Alpha"=0.0, "Alpha Blending Enabled"=FALSE, "Colour"=131841}, {"Vertex 1"={"Position"={"x"=527.4663, "y"=105.9543, "z"=0.9882486}, "UV"={"u"=0.0, "v"=0.0}, "Colour"=12517256}, "Vertex 2"={"Position"={"x"=539.10596, "y"=105.47977, "z"=0.9880842}, "UV"={"u"=0.0, "v"=0.0}, "Colour"=12517256}, "Vertex 3"={"Position"={"x"=546.60223, "y"=113.55681, "z"=0.98858106}, "UV"={"u"=0.0, "v"=0.0}, "Colour"=12517256}, "Alpha"=0.0, "Alpha Blending Enabled"=FALSE, "Colour"=131841}, {"Vertex 1"={"Position"={"x"=506.44025, "y"=404.4099, "z"=0.98854554}, "UV"={"u"=0.0, "v"=0.0}, "Colour"=12517256}, "Vertex 2"={"Position"={"x"=518.25006, "y"=402.50375, "z"=0.98837876}, "UV"={"u"=0.0, "v"=0.0}, "Colour"=12517256}, "Vertex 3"={"Position"={"x"=507.2441, "y"=405.96255, "z"=0.9879849}, "UV"={"u"=0.0, "v"=0.0}, "Colour"=12517256}, "Alpha"=0.0, "Alpha Blending Enabled"=FALSE, "Colour"=10014061}, {"Vertex 1"={"Position"={"x"=241.36343, "y"=397.0934, "z"=0.9884605}, "UV"={"u"=0.0, "v"=0.0}, "Colour"=12517256}, "Vertex 2"={"Position"={"x"=243.93146, "y"=400.19006, "z"=0.9884862}, "UV"={"u"=0.0, "v"=0.0}, "Colour"=12517256}, "Vertex 3"={"Position"={"x"=251.49637, "y"=404.82367, "z"=0.9879514}, "UV"={"u"=0.0, "v"=0.0}, "Colour"=12517256}, "Alpha"=0.0, "Alpha Blending Enabled"=FALSE, "Colour"=9025634}, {"Vertex 1"={"Position"={"x"=245.69356, "y"=114.66924, "z"=0.9885038}, "UV"={"u"=0.0, "v"=0.0}, "Colour"=12517256}, "Vertex 2"={"Position"={"x"=241.30443, "y"=116.502, "z"=0.9884599}, "UV"={"u"=0.0, "v"=0.0}, "Colour"=12517256}, "Vertex 3"={"Position"={"x"=248.879, "y"=107.86597, "z"=0.98791444}, "UV"={"u"=0.0, "v"=0.0}, "Colour"=12517256}, "Alpha"=0.0, "Alpha Blending Enabled"=FALSE, "Colour"=131841}, {"Vertex 1"={"Position"={"x"=425.6105, "y"=412.44833, "z"=0.98858166}, "UV"={"u"=0.0, "v"=0.0}, "Colour"=12517256}, "Vertex 2"={"Position"={"x"=432.43652, "y"=413.4734, "z"=0.9881905}, "UV"={"u"=0.0, "v"=0.0}, "Colour"=12517256}, "Vertex 3"={"Position"={"x"=416.8047, "y"=414.309, "z"=0.98810315}, "UV"={"u"=0.0, "v"=0.0}, "Colour"=12517256}, "Alpha"=0.0, "Alpha Blending Enabled"=FALSE, "Colour"=10013805}, {"Vertex 1"={"Position"={"x"=593.1241, "y"=145.61699, "z"=0.9881152}, 
